vi "Skyline Send Waveform Tags.vi"(8 "error in (no error)":errorcluster, 9 "Keywords":string[](array[string]), 10 "Decimate to single value":bool=TRUE, 11 "data in":waveform(dbl)[](array[waveform])) -> (0 "error out":errorcluster, 3 "data out":waveform(dbl)[](array[waveform]))   [LabVIEW 2016]
uses:
  <vilib>/TagLibrary/DataType.ctl
  <vilib>/TagLibrary/TagLibrary.lvlib
  <resource>/objmgr/niTag.rc
  <vilib>/TagLibrary/Create Tag (Double).vi
  <vilib>/TagLibrary/Close Tag (Single).vi
  <vilib>/TagLibrary/Write (Waveform).vi
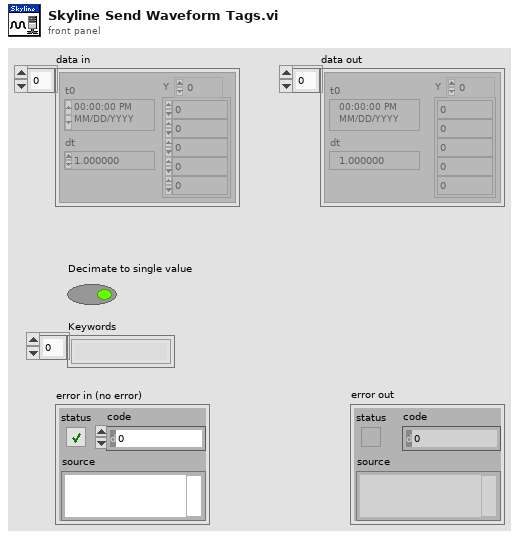
[diagram p1: front panel]
types:
  T1 = typedef "TagLibrary.lvlib/DataType.ctl" = enum32{"Double", "Integer", "String"}
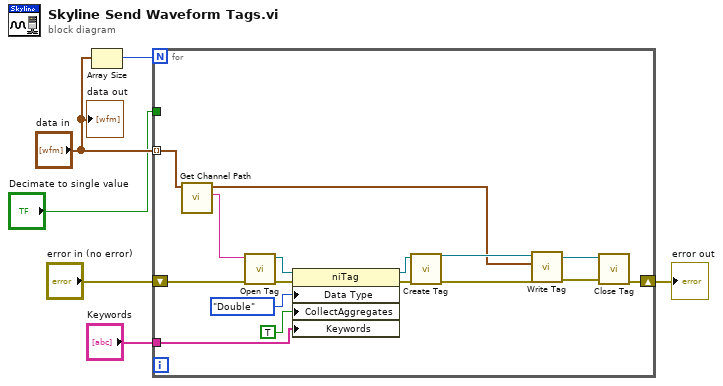
[diagram p0: block diagram]
diagram:
  n1 = Array Size(array="data in") -> (size(s)=w5:i32)
  n2 = for {
    N: w5 -> [_]
    tunnel: "data in" -> [w22] mode=indexing
    shift-right: [w17] -> w3
    shift-left: "error in (no error)" -> [w16]
    tunnel: "Decimate to single value" -> [_]
    tunnel: "Keywords" -> [w15]
    n3 = call "Get Channel Path.vi"("Waveform"=w22) -> ("channel path"=w8:string, "Waveform out"=w7:waveform(dbl))  [unwired: 9 in]
    n4 = call <vilib>:"Open Tag.vi"("error in (no error)"=w16, "tag path"=w8) -> ("error out"=w21:errorcluster, "tag reference out"=w18:refnum<k21>)  [unwired: 8 in]
    n5 = property class="niTag"(reference=w18, error in=w21, "Data Type"=DataType."Double", "CollectAggregates"=TRUE, "Keywords"=w15) -> (reference out=w13:refnum<k21>, error out=w14:errorcluster)
    n6 = call-poly <vilib>:"Create Tag.vi"("error in (no error)"=w14, "tag reference in"=w13) -> ("error out"=w10:errorcluster, "tag reference out"=w11:refnum<k21>)  [unwired: 8 in]
    n7 = call-poly <vilib>:"Write Tag.vi"("error in (no error)"=w10, "Waveform"=w7, "tag reference in"=w11) -> ("error out"=w9:errorcluster, "tag reference out"=w12:refnum<k21>)  [unwired: 7 in]
    n8 = call-poly <vilib>:"Close Tag.vi"("error in (no error)"=w9, "tag reference"=w12) -> ("error out"=w17:errorcluster)  [unwired: 9 in]
  }
  "error out" <- w3
  "data out" <- "data in"
